vi "Global_Rating.vi"() -> ()   [LabVIEW 2020]
panel:
  out "output_rating":dbl
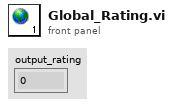
[diagram p1: front panel]
diagram:
